vi "MyNewSample.vi"() -> ()   [LabVIEW 2012]
panel:
  out "Detector\nTemperature":dbl
  in  "Enter the Detector\nTemperature (C)":dbl
  out "Spectrum of the first Spectrometer":cluster{"Y":dbl[], "Y":dbl[]}[](graph)
  in  "stop":bool
  in  "Enter the \nInetegration Time (µs)":i32
  in  "Start":bool=TRUE
  out "Number of \nSpectrometers":i32
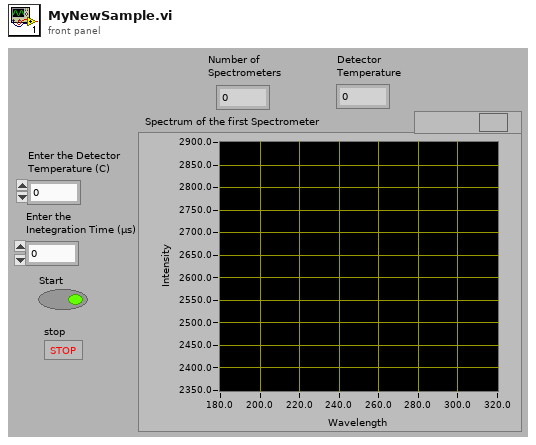
[diagram p1: front panel]
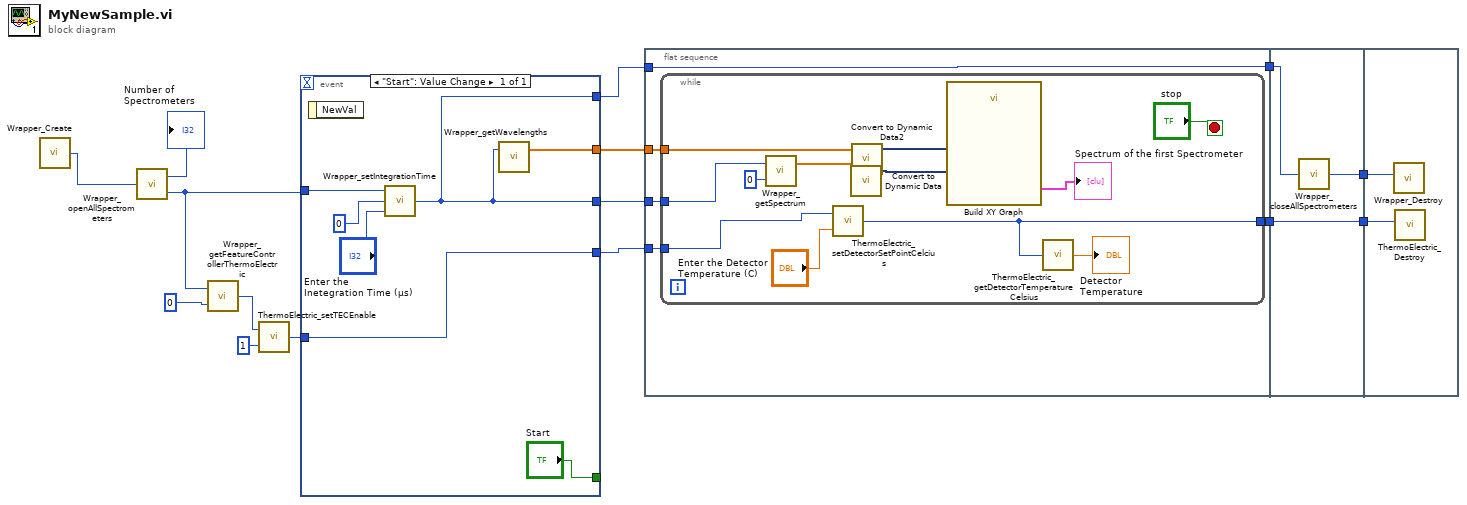
[diagram p0: block diagram]
diagram:
  n1 = call <instrlib>:"Wrapper_Create.vi"() -> ("Wrapper"=w15:u64)
  n2 = call <instrlib>:"Wrapper_openAllSpectrometers.vi"("Wrapper In"=w15) -> ("Number of Spectrometers"=→"Number of \nSpectrometers":i32, "Wrapper Out"=w8:u64)
  n3 = call <instrlib>:"Wrapper_getFeatureControllerThermoElectric.vi"("Index"=0, "Wrapper"=w8) -> ("ThermoElectric"=w6:u64)
  n4 = call <instrlib>:"ThermoElectric_setTECEnable.vi"("Enable"=u8 1, "ThermoElectric In"=w6) -> ("ThermoElectric Out"=w4:u64)
  n5 = event shown="[0] \"Start\": Value Change" {
    selector: _ -> [_]
    dyn-events: _ -> [_]
    timeout: _ -> [_]
    tunnel: ["Start"] -> _
    tunnel: w8 -> [w19]
    tunnel: [w17] -> w13
    tunnel: [w18] -> w12
    tunnel: [w17] -> w10
    tunnel: w4 -> [w16]
    tunnel: [w16] -> w3
    event "Start": Value Change {
      n6 = event-data() -> ()  [unwired: 1 in, 1 out]
      n7 = call <instrlib>:"Wrapper_setIntegrationTime.vi"("Integration Time"="Enter the \nInetegration Time (µs)", "Index"=0, "Wrapper In"=w19) -> ("Wrapper Out"=w17:u64)
      n8 = call <instrlib>:"Wrapper_getWavelengths.vi"("Wrapper"=w17) -> ("WL Values"=w18:dbl[])  [unwired: 1 in, 1 out]
    }
  }
  n9 = flat-sequence {
    tunnel: w13 -> [w27]
    tunnel: w12 -> [w26]
    tunnel: [w25] -> w11
    tunnel: w10 -> [w25]
    tunnel: w3 -> [w24]
    tunnel: [w23] -> w1
    tunnel: w11 -> [w41]
    tunnel: [w42] -> w9
    tunnel: [w40] -> w2
    tunnel: w1 -> [w40]
    tunnel: w9 -> [w44]
    tunnel: w2 -> [w43]
    frame #0 {
      n10 = while {
        tunnel: w27 -> [w39]
        tunnel: w26 -> [w33]
        tunnel: w24 -> [w30]
        tunnel: [w28] -> w23
        stop <- "stop" stop-if-true
        n11 = call <instrlib>:"Wrapper_getSpectrum.vi"("Index"=0, "Wrapper"=w39) -> ("Spectrum Values"=w35:dbl[])  [unwired: 1 out]
        n12 = call <instrlib>:"ThermoElectric_setDetectorSetPointCelcius.vi"("Temperature"="Enter the Detector\nTemperature (C)", "ThermoElectric In"=w30) -> ("ThermoElectric Out"=w28:u64)
        n13 = call "Convert to Dynamic Data"("Array"=w35) -> ("Dynamic Data Type"=w34:dynamicdata)  [unwired: 3 in]
        n14 = call "Convert to Dynamic Data2"("Array"=w33) -> ("Dynamic Data Type"=w32:dynamicdata)  [unwired: 3 in]
        n15 = call "Build XY Graph"("Y Input"=w34, "X Input"=w32) -> ("XY Graph"=→"Spectrum of the first Spectrometer":cluster{"Y":dbl[], "Y":dbl[]}[])  [unwired: 8 in, 1 out]
        n16 = call <instrlib>:"ThermoElectric_getDetectorTemperatureCelsius.vi"("ThermoElectric"=w28) -> ("Temperature"=→"Detector\nTemperature":dbl)
      }
    }
    frame #1 {
      n17 = call <instrlib>:"Wrapper_closeAllSpectrometers.vi"("Wrapper In"=w41) -> ("Wrapper Out"=w42:u64)
    }
    frame #2 {
      n18 = call <instrlib>:"Wrapper_Destroy.vi"("Wrapper"=w44) -> ()
      n19 = call <instrlib>:"ThermoElectric_Destroy.vi"("ThermoElectric"=w43) -> ()
    }
  }
